vi "QueryNTPparse.vi"(0 "IP Address of NIST Server":string="132.163.4.102", 1 "error in (no error)":errorcluster) -> (2 "NTP Time (server time)":u64, 3 "time stamp UTC":timestamp, 4 "error out":errorcluster)   [LabVIEW 2012]
panel:
  out "NTP time (UTC)":i64
  out "time stamp NTP (UTC)":timestamp
  out "time stamp":timestamp
  out "raw data":string
  # "This is a first draft to query an NTP server (proof of concept).\nhttp://forums.ni.com/ni/board/message?board.id=170&message.id=458949&jump=true"
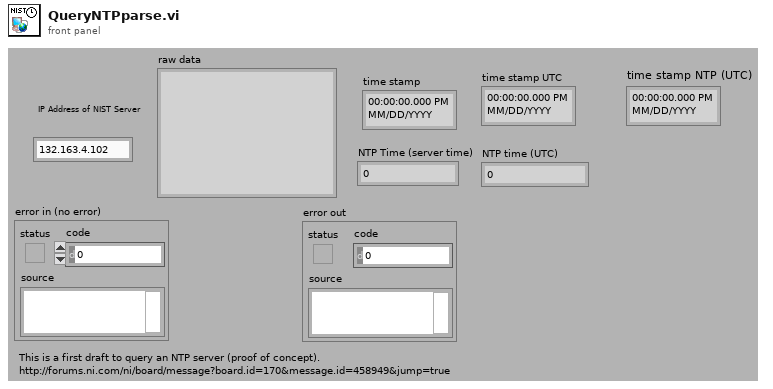
[diagram p1: front panel]
types:
  T1 = cluster{"LI|VM|Mode":u8, "Stratum":u8, "Poll":u8, "Precision":u8, "Root Delay":u32, "Root Dispersion":u32, "Reference Identifier":u32, "Reference Timestamp":fxp<+,64,32>, "Originate Timestamp":fxp<+,64,32>, "Receive Timestamp":fxp<+,64,32>, "Transmit Timestamp":fxp<+,64,32>, "Key Identifier":u32, "Message Digest-1":u64, "Message Digest-2":u64}
  T2 = typedef "LVDateTimeRec.ctl" = cluster{"fractional second":dbl, "second":i32, "minute":i32, "hour":i32, "day of month":i32, "month":i32, "year":i32, "day of week":i32, "day of year":i32, "DST":i32}
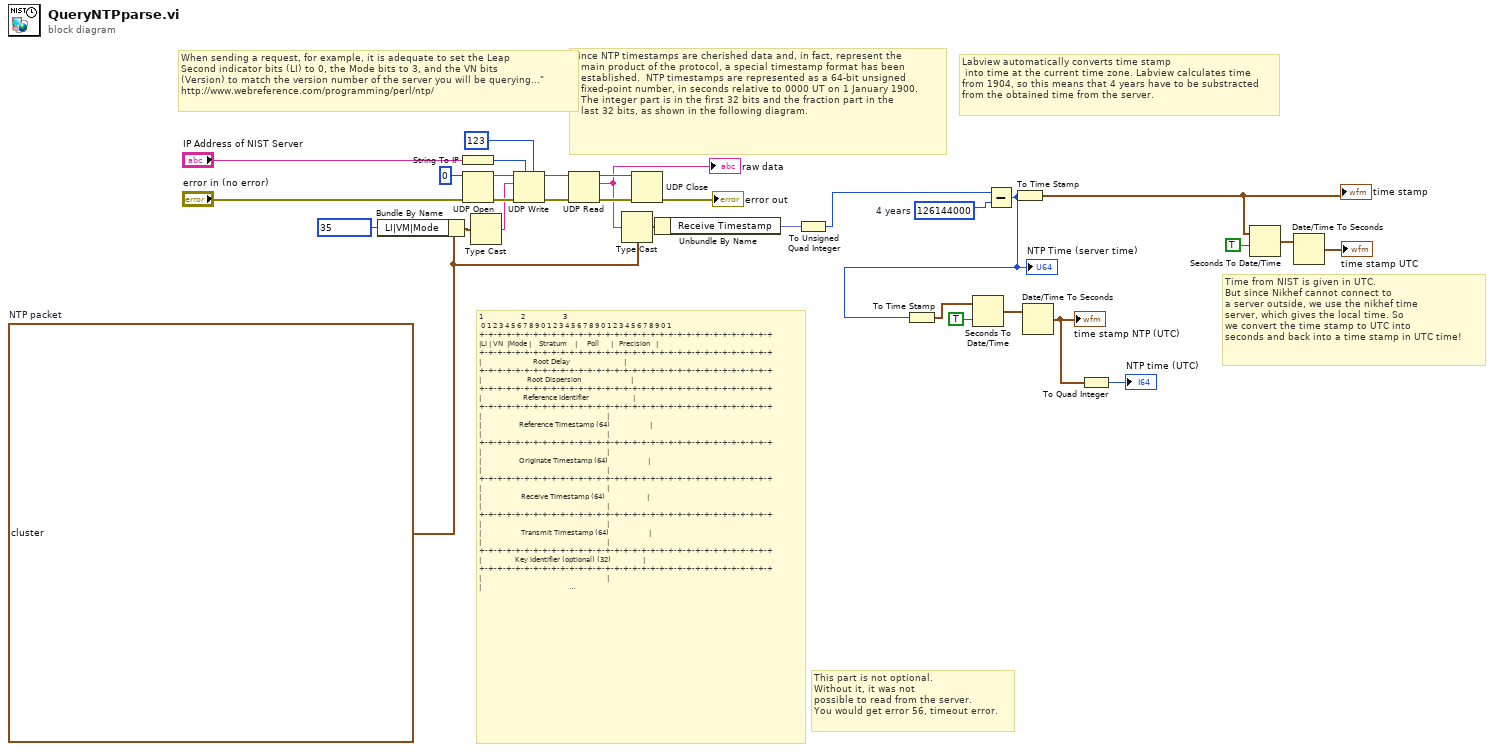
[diagram p0: block diagram]
diagram:
  w12 = T1 {"LI|VM|Mode"=0, "Stratum"=0, "Poll"=0, "Precision"=0, "Root Delay"=0, "Root Dispersion"=0, "Reference Identifier"=0, "Reference Timestamp"=0.0, "Originate Timestamp"=0.0, "Receive Timestamp"=0.0, "Transmit Timestamp"=0.0, "Key Identifier"=0, "Message Digest-1"=0, "Message Digest-2"=0}  # NTP packet
  w13 = u64 126144000  # 4 years
  # "This part is not optional.\nWithout it, it was not \npossible to read from the server.\nYou would get error 56, timeout error."
  # "Labview automatically converts time stamp\n into time at the current time zone. Labview calculates time\nfrom 1904, so this means that 4 years have to be substracted\nfrom the obtained time from the server."
  # "Time from NIST is given in UTC.\nBut since Nikhef cannot connect to\na server outside, we use the nikhef time \nserver, which gives the local time. So\nwe convert the time stamp to UTC into\nseconds and back into a time stamp in UTC time!"
  # "Since NTP timestamps are cherished data and, in fact, represent the\n   main product of the protocol, a special timestamp format has been\n   established.  NTP timestamps are represented as a 64-bit unsigned\n   fixed-point number, in seconds relative to 0000 UT on 1 January 1900.\n   The integer part is in the first 32 bits and the fraction part in the\n   last 32 bits, as shown in the following diagram."
  # "When sending a request, for example, it is adequate to set the Leap\nSecond indicator bits (LI) to 0, the Mode bits to 3, and the VN bits\n(Version) to match the version number of the server you will be querying...\"\nhttp://www.webreference.com/programming/perl/ntp/"
  # "1                   2                   3\n 0 1 2 3 4 5 6 7 8 9 0 1 2 3 4 5 6 7 8 9 0 1 2 3 4 5 6 7 8 9 0 1\n+-+-+-+-+-+-+-+-+-+-+-+-+-+-+-+-+-+-+-+-+-+-+-+-+-+-+-+-+-+-+-+-+\n|LI | VN  |Mode |    Stratum    |     Poll      |   Precision   |\n+-+-+-+-+-+-+-+-+-+-+-+-+-+-+-+-+-+-+-+-+-+-+-+-+-+-+-+-+-+-+-+-+\n|                          Root Delay                           |\n+-+-+-+-+-+-+-+-+-+-+-+-+-+-+-+-+-+-+-+-+-+-+-+-+-+-+-+-+-+-+-+-+\n|                       Root Dispersion                         |\n+-+-+-+-+-+-+-+-+-+-+-+-+-+-+-+-+-+-+-+-+-+-+-+-+-+-+-+-+-+-+-+-+\n|                     Reference Identifier                      |\n+-+-+-+-+-+-+-+-+-+-+-+-+-+-+-+-+-+-+-+-+-+-+-+-+-+-+-+-+-+-+-+-+\n|                                                               |\n|                   Reference Timestamp (64)                    |\n|                                                               |\n+-+-+-+-+-+-+-+-+-+-+-+-+-+-+-+-+-+-+-+-+-+-+-+-+-+-+-+-+-+-+-+-+\n|                                                               |\n|                   Originate Timestamp (64)                    |\n|                                                               |\n+-+-+-+-+-+-+-+-+-+-+-+-+-+-+-+-+-+-+-+-+-+-+-+-+-+-+-+-+-+-+-+-+\n|                                                               |\n|                    Receive Timestamp (64)                     |\n|                                                               |\n+-+-+-+-+-+-+-+-+-+-+-+-+-+-+-+-+-+-+-+-+-+-+-+-+-+-+-+-+-+-+-+-+\n|                                                               |\n|                    Transmit Timestamp (64)                    |\n|                                                               |\n+-+-+-+-+-+-+-+-+-+-+-+-+-+-+-+-+-+-+-+-+-+-+-+-+-+-+-+-+-+-+-+-+\n|                 Key Identifier (optional) (32)                |\n+-+-+-+-+-+-+-+-+-+-+-+-+-+-+-+-+-+-+-+-+-+-+-+-+-+-+-+-+-+-+-+-+\n|                                                               |\n|                                                               |\n|                 Message Digest (optional) (128)               |\n|                                                               |\n|                                                               |\n+-+-+-+-+-+-+-+-+-+-+-+-+-+-+-+-+-+-+-+-+-+-+-+-+-+-+-+-+-+-+-+-+"
  n1 = Bundle By Name(cluster=w12, "LI|VM|Mode"=u8 35) -> (w14:T1)
  n2 = String To IP(1:"IP Address of NIST Server") -> (0:w26:u32)
  n3 = UDP Open(8:"error in (no error)", 11:u16 0 ("port")) -> (port=w28:refnum<k16>, 0:w25:errorcluster)  [unwired: 3 in, 1 out]
  n4 = Type Cast(x=w14) -> (*(type *) &x=w21:string)  [unwired: 1 in]
  n5 = UDP Write(address=w26, port or service name=u16 123, connection ID=w28, data in=w21, 8:w25) -> (error out=w24:errorcluster, 3:w29:refnum<k16>)  [unwired: 1 in]
  n6 = UDP Read(connection ID=w29, 8:w24) -> (data out=w18:string, error out=w31:errorcluster, 3:w30:refnum<k16>)  [unwired: 2 in, 2 out]
  "raw data" <- w18
  n7 = Type Cast(type=w12, x=w18) -> (*(type *) &x=w17:T1)
  n8 = UDP Close(connection ID=w30, 8:w31) -> (error out=→"error out":errorcluster)  [unwired: 1 out]
  n9 = Unbundle By Name(w17) -> ("Receive Timestamp"=w16:fxp<+,64,32>)
  n10 = To Unsigned Quad Integer(1:w16) -> (0:w5:u64)
  n11 = Subtract(x=w5, y=w13) -> (x-y=w2:u64)
  "NTP Time (server time)" <- w2
  n12 = To Time Stamp(1:w2) -> (0:w4:timestamp)
  n13 = Seconds To Date/Time(time stamp (now)=w4, to UTC (F)=TRUE) -> (date time rec=w6:T2)
  n14 = To Time Stamp(1:w2) -> (0:w9:timestamp)
  "time stamp" <- w9
  n15 = Date/Time To Seconds(2:w6) -> (0:w3:timestamp)  [unwired: 1 in]
  "time stamp NTP (UTC)" <- w3
  n16 = To Quad Integer(1:w3) -> (0:→"NTP time (UTC)":i64)
  n17 = Seconds To Date/Time(time stamp (now)=w9, to UTC (F)=TRUE) -> (date time rec=w11:T2)
  n18 = Date/Time To Seconds(2:w11) -> (0:→"time stamp UTC":timestamp)  [unwired: 1 in]
